vi "Delete EST Loops.vi"(8 "error in (no error)":errorcluster, 11 "Main Sequence in":refnum<class "Main Sequence.lvclass">) -> (0 "error out":errorcluster, 3 "Main Sequence out":refnum<class "Main Sequence.lvclass">)   [LabVIEW 2015, in "Main Sequence.lvclass"]
uses:
  Main Sequence.lvclass
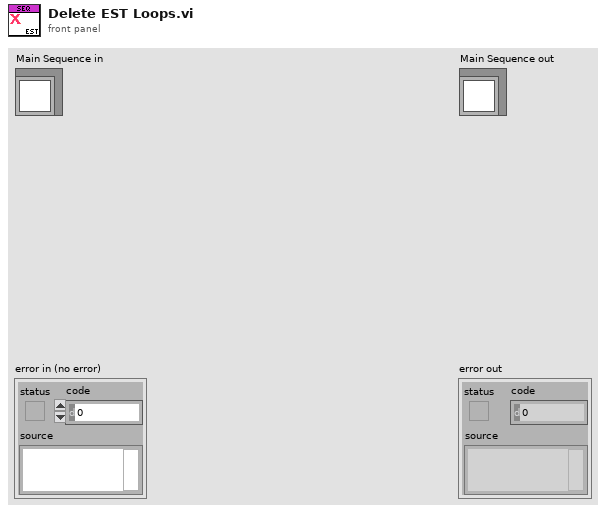
[diagram p1: front panel]
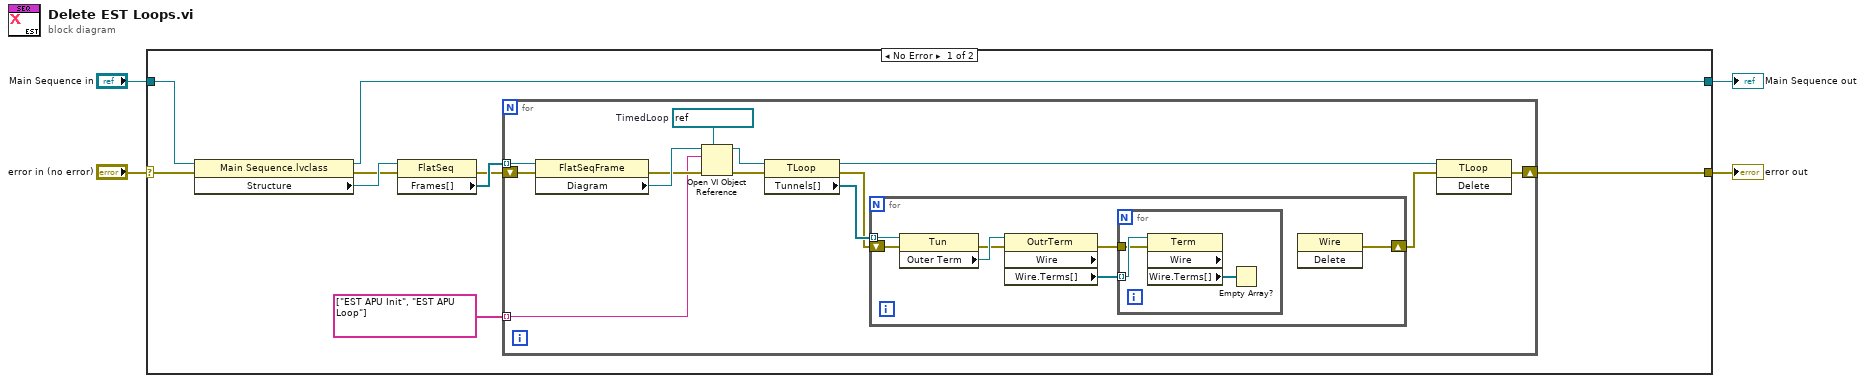
[diagram p0: block diagram]
diagram:
  n1 = case shown="No Error" "error in (no error)" {
    selector: "error in (no error)" -> [w11 w38]
    tunnel: [w5 w38] -> w3
    tunnel: [w12 w37] -> w1
    tunnel: "Main Sequence in" -> [w13 w37]
    frame No Error {
      n2 = property class="Main Sequence.lvclass"(reference=w13, error in=w11) -> (reference out=w12:refnum<class "Main Sequence.lvclass">, error out=w9:errorcluster, "Structure"=w10:refnum<vi>)
      n3 = property class="FlatSeq"(reference=w10, error in=w9) -> (error out=w7:errorcluster, "Frames[]"=w8:refnum<vi>[])  [unwired: 1 out]
      n4 = for {
        tunnel: w8 -> [w25] mode=indexing
        shift-right: [w20] -> w5
        shift-left: w7 -> [w26]
        tunnel: string[] ["EST APU Init", "EST APU Loop"] -> [w21] mode=indexing
        w23 = refnum<vi> refnum  # TimedLoop
        n5 = property class="FlatSeqFrame"(reference=w25, error in=w26) -> (error out=w22:errorcluster, "Diagram"=w24:refnum<vi>)  [unwired: 1 out]
        n6 = Open VI Object Reference(7:w23, 8:w22, 10:w21, 11:w24) -> (0:w18:errorcluster, 3:w19:refnum<vi>)
        n7 = property class="TLoop"(reference=w19, error in=w18) -> (reference out=w17:refnum<vi>, error out=w15:errorcluster, "Tunnels[]"=w16:refnum<vi>[])
        n8 = for {
          tunnel: w16 -> [w33] mode=indexing
          shift-right: [w29] -> w14
          shift-left: w15 -> [w31]
          n9 = property class="Tun"(reference=w33, error in=w31) -> (error out=w30:errorcluster, "Outer Term"=w32:refnum<vi>)  [unwired: 1 out]
          n10 = property class="OutrTerm" props=["Wire", "Wire", "Terms[]"](reference=w32, error in=w30) -> (error out=w27:errorcluster, "Wire.Terms[]"=w28:refnum<vi>[])  [unwired: 2 out]
          n11 = for {
            tunnel: w28 -> [w36] mode=indexing
            tunnel: w27 -> [w35]
            n12 = property class="Term" props=["Wire", "Wire", "Terms[]"](reference=w36, error in=w35) -> ("Wire.Terms[]"=w34:refnum<vi>[])  [unwired: 3 out]
            n13 = Empty Array?(array=w34) -> ()  [unwired: 1 out]
          }
          n14 = invoke class="Wire" method="Delete"() -> (error out=w29:errorcluster)  [unwired: 3 in, 2 out]
        }
        n15 = invoke class="TLoop" method="Delete"(reference=w17, error in=w14) -> (error out=w20:errorcluster)  [unwired: 1 in, 2 out]
      }
    }
    frame Error {
    }
  }
  "error out" <- w3
  "Main Sequence out" <- w1
